vi "XYZ Ultrasonic Scanning Software v1.3 (Data-Acq-Osc).vi"() -> ()   [LabVIEW 2020]
doc: "Allows the user to trigger an A-Scan reading from the oscilloscope and check the connection with the machine."
uses:
  <instrlib>/LeCroy Wave Series/LeCroy Wave Series.lvlib
panel:
  in  "Tab Control":T1(tab)
  in  "VISA Resource Name (Osc. Model Used)":refnum<visa-resource-name>
  out "Succesful Osc Connection":bool=TRUE
  in  "Check Osc Connection":bool
  out "A-Scan":waveform(dbl)(graph)
  in  "Acquire A-Scan":bool
  in  "File Format":T2(radio)
  in  "VISA resource name":refnum<visa-resource-name>
  in  "Source (0: Channel 1)":u16(ring) items=["Channel 1", "Channel 2", "Channel 3", "Channel 4", "Memory 1", "Memory 2", "Memory 3", "Memory 4", "Function 1", "Function 2", "Function 3", "Function 4", "Function 5", "Function 6", "Function 7", "Function 8"]
  in  "Folder to Save A-Scan":path
  in  "File Name for A-Scan":string
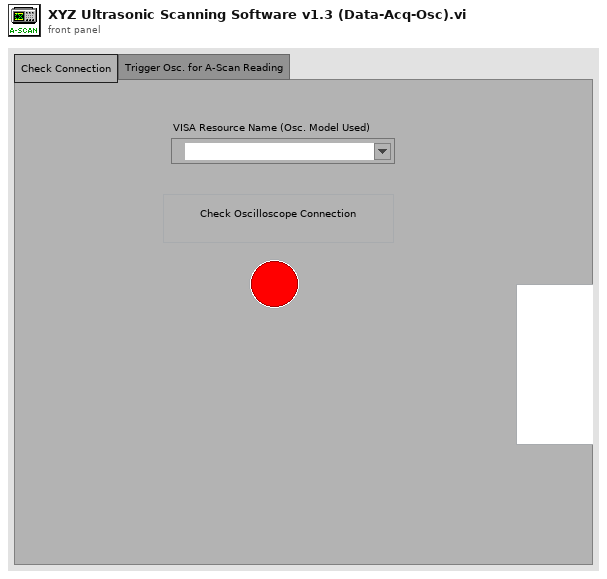
[diagram p1: front panel]
types:
  T1 = enum32{"Check Connection", "Trigger Osc. for A-Scan Reading"}
  T2 = enum32{"No Selection", "Do Not Save", "ASCII", "CSV", "MATLAB"}
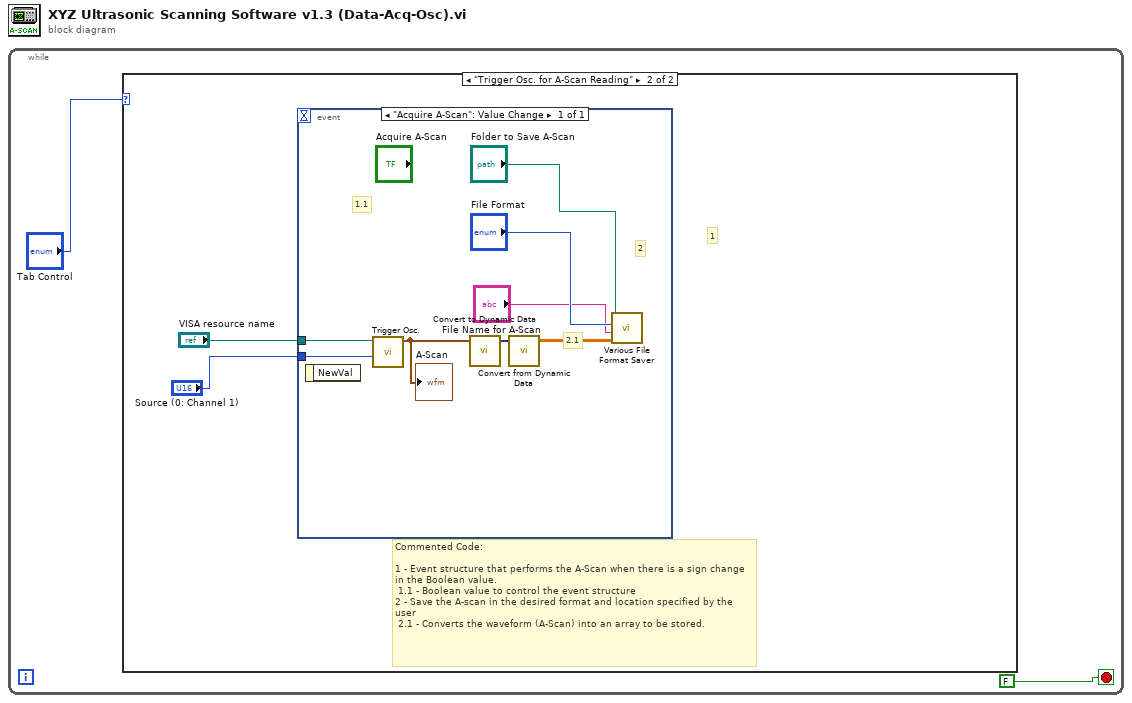
[diagram p0: block diagram]
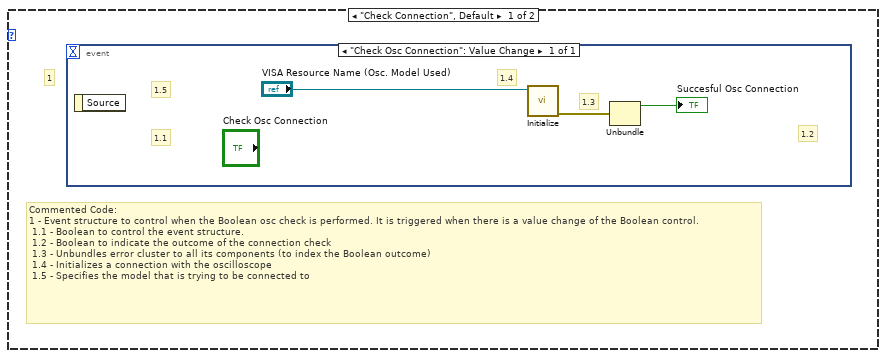
[diagram p2: hidden frame]
diagram:
  n1 = while {
    stop <- FALSE stop-if-true
    n2 = case shown="\"Trigger Osc. for A-Scan Reading\"" "Tab Control" {
      frame "Check Connection", Default {
        # "1"
        # "Commented Code:\n1 - Event structure to control when the Boolean osc check is performed. It is triggered when there is a value change of the Boolean control. \n 1.1 - Boolean to control the event structure.\n 1.2 - Boolean to indicate the outcome of the connection check\n 1.3 - Unbundles error cluster to all its components (to index the Boolean outcome)\n 1.4 - Initializes a connection with the oscilloscope\n 1.5 - Specifies the model that is trying to be connected to"
        n3 = event shown="[0] \"Check Osc Connection\": Value Change" {
          selector: _ -> [_]
          dyn-events: _ -> [_]
          timeout: _ -> [_]
          event "Check Osc Connection": Value Change {
            # "1.5"
            # "1.4"
            # "1.3"
            # "1.2"
            # "1.1"
            n4 = event-data() -> ()  [unwired: 1 in, 1 out]
            n5 = call <instrlib>:"Initialize.vi"("VISA resource name"="VISA Resource Name (Osc. Model Used)") -> ("error out"=w5:errorcluster)  [unwired: 9 in, 1 out]
            n6 = Unbundle(w5) -> ("status"=→"Succesful Osc Connection":bool)  [unwired: 2 out]
          }
        }
      }
      frame "Trigger Osc. for A-Scan Reading" {
        # "1"
        # "Commented Code:\n\n1 - Event structure that performs the A-Scan when there is a sign change in the Boolean value.\n 1.1 - Boolean value to control the event structure\n2 - Save the A-scan in the desired format and location specified by the user\n 2.1 - Converts the waveform (A-Scan) into an array to be stored."
        n7 = event shown="[0] \"Acquire A-Scan\": Value Change" {
          selector: _ -> [_]
          dyn-events: _ -> [_]
          timeout: _ -> [_]
          tunnel: "VISA resource name" -> [w15]
          tunnel: "Source (0: Channel 1)" -> [w14]
          event "Acquire A-Scan": Value Change {
            # "2.1"
            # "2"
            # "1.1"
            n8 = event-data() -> ()  [unwired: 1 in, 1 out]
            n9 = call "Trigger Osc..vi"("Source (0: Channel 1)"=w14, "VISA resource name"=w15) -> ("Waveform Data"=w13:waveform(dbl))  [unwired: 9 in]
            "A-Scan" <- w13
            n10 = call "Convert to Dynamic Data"("Waveform"=w13) -> ("Dynamic Data Type"=w12:dynamicdata)  [unwired: 3 in]
            n11 = call "Convert from Dynamic Data"("Dynamic Data Type"=w12) -> ("Array"=w11:dbl[][])  [unwired: 3 in]
            n12 = call "Various File Format Saver.vi"("Incoming Data to be Saved"=w11, "File Name"="File Name for A-Scan", "File Format"="File Format", "Folder to Save Data"="Folder to Save A-Scan") -> ()  [unwired: 8 in]
          }
        }
      }
    }
  }
